vi "Working Point 2 Selection Dialog.vi"(7 "DisplayFilter":u8(ring)=7 items=["K_CHAN_R", "K_CHAN_W", "K_CHAN_RW", "K_CHAN_VOLT", "K_CHAN_FAULT", "K_ALL", "K_CUSTOM", "K_CHAN_R_VIS", "K_CHAN_W_VIS", "K_CHAN_RW_VIS", "K_CHAN_VOLT_VIS", "K_CHAN_FAULT_VIS"], 8 "error in (no error)":errorcluster, 9 "NIVS.System Definition Root":refnum<k24>, 10 "NodePaths":string[](array[string])) -> (0 "error out":errorcluster, 2 "Selected NodePaths":string[](array[string]))   [LabVIEW 2011]
doc: "Use this template to create a dialog box with event handling."
uses:
  NationalInstruments.VeriStand.SystemStorageUI
  NationalInstruments.VeriStand.SystemStorage
  <vilib>/NI Veristand/UI Controls/Single Node Browser/Net Event Data.ctl
  <vilib>/NI Veristand/UI Controls/Single Node Browser/Net Event.ctl
  <vilib>/NI Veristand/UI Controls/Single Node Browser/NI_VS UI Single Node Browser.lvlib
panel:
  in  "Y Value":refnum<k24>(container)
  in  "Cancel":bool
  in  "Ok":bool
  in  "X Index":refnum<k24>(container)
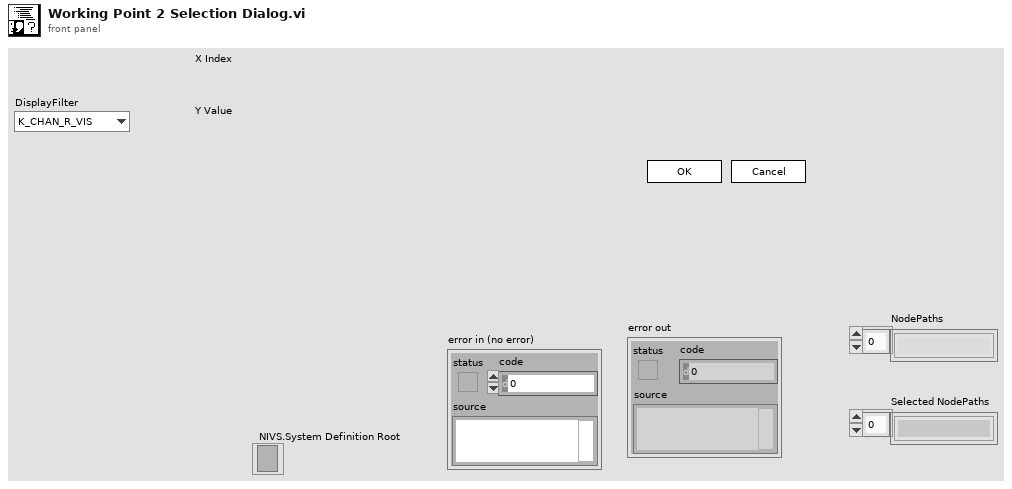
[diagram p1: front panel]
types:
  T1 = typedef "NI_VS UI Single Node Browser.lvlib/Callback Type.ctl" = cluster{"Net Callbacks":refnum<k27>[], "Event":refnum<user-event>}
  T2 = typedef "NI_VS UI Single Node Browser.lvlib/Node Ref.ctl" = refnum<k24>
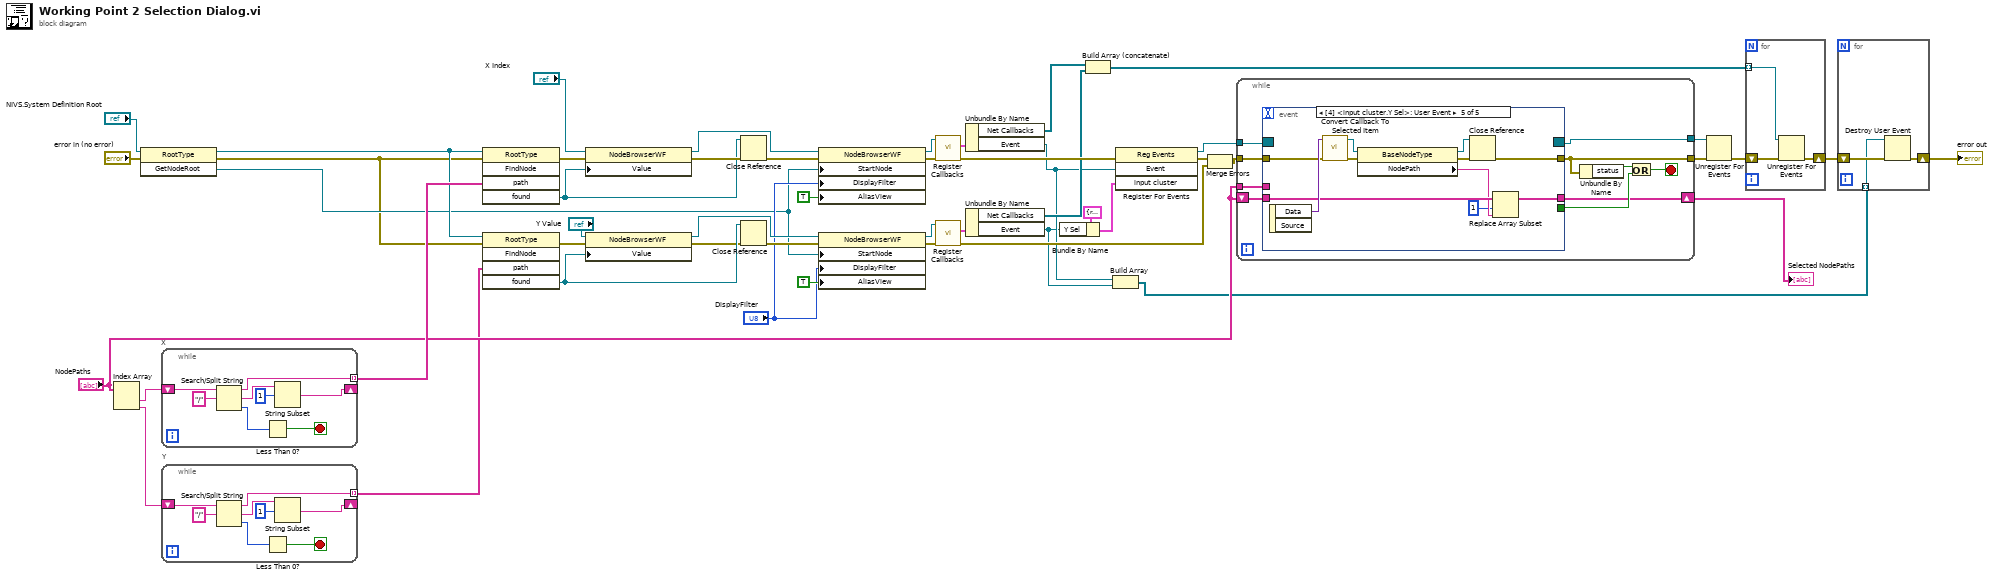
[diagram p0: block diagram]
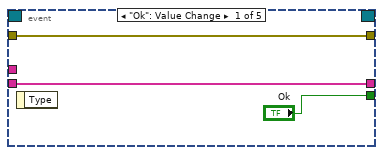
[diagram p2: hidden frame]
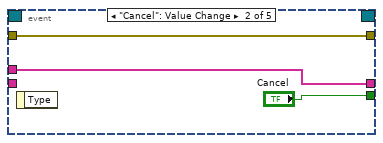
[diagram p3: hidden frame]
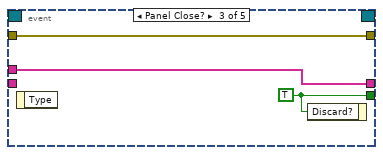
[diagram p4: hidden frame]
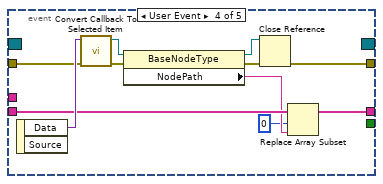
[diagram p5: hidden frame]
diagram:
  n1 = Index Array(array="NodePaths") -> (element #1=w30:string, element #2=w29:string)  [unwired: 2 in]
  n2 = invoke class="RootType" method="GetNodeRoot"(reference="NIVS.System Definition Root", error in="error in (no error)") -> (reference out=w18:refnum<k24>, error out=w14:errorcluster, "GetNodeRoot"=w15:refnum<k24>)  [unwired: 1 in]
  n3 = while "X" {
    tunnel: [w54] -> w36 mode=indexing
    shift-right: [w52] -> _
    shift-left: w30 -> [w58]
    stop <- w55 stop-if-true
    n4 = Search/Split String(string=w58, search string/char (-)="/") -> (substring before match=w54:string, match + rest of string=w53:string, offset of match=w56:i32)  [unwired: 1 in]
    n5 = Less Than 0?(x=w56) -> (x < 0?=w55:bool)
    n6 = String Subset(string=w53, offset (0)=1) -> (substring=w52:string)  [unwired: 1 in]
  }
  n7 = while "Y" {
    tunnel: [w62] -> w13 mode=indexing
    shift-right: [w60] -> _
    shift-left: w29 -> [w66]
    stop <- w63 stop-if-true
    n8 = Search/Split String(string=w66, search string/char (-)="/") -> (substring before match=w62:string, match + rest of string=w61:string, offset of match=w64:i32)  [unwired: 1 in]
    n9 = Less Than 0?(x=w64) -> (x < 0?=w63:bool)
    n10 = String Subset(string=w61, offset (0)=1) -> (substring=w60:string)  [unwired: 1 in]
  }
  n11 = invoke class="RootType" method="FindNode"(reference=w18, error in=w14, "path"=w36) -> (error out=w42:errorcluster, "found"=w37:refnum<k24>)  [unwired: 2 in, 3 out]
  n12 = invoke class="RootType" method="FindNode"(reference=w18, error in=w14, "path"=w13) -> (error out=w23:errorcluster, "found"=w26:refnum<k24>)  [unwired: 2 in, 3 out]
  n13 = property class="NodeBrowserWF"(reference="X Index", error in=w42, "Value"=w37) -> (reference out=w31:refnum<k24>, error out=w39:errorcluster)
  n14 = property class="NodeBrowserWF"(reference="Y Value", error in=w23, "Value"=w26) -> (reference out=w27:refnum<k24>, error out=w24:errorcluster)
  n15 = Close Reference(reference=w37, error in (no error)=w39) -> (error out=w38:errorcluster)
  n16 = Close Reference(reference=w26, error in (no error)=w24) -> (error out=w25:errorcluster)
  n17 = property class="NodeBrowserWF"(reference=w31, error in=w38, "StartNode"=w15, "DisplayFilter"="DisplayFilter", "AliasView"=TRUE) -> (reference out=w44:refnum<k24>, error out=w45:errorcluster)
  n18 = property class="NodeBrowserWF"(reference=w27, error in=w25, "StartNode"=w15, "DisplayFilter"="DisplayFilter", "AliasView"=TRUE) -> (reference out=w21:refnum<k24>, error out=w20:errorcluster)
  n19 = call <vilib>:"Register Callbacks.vi"("error in (no error)"=w45, "Single Node Browser"=w44) -> ("error out"=w50:errorcluster, "Callbacks"=w46:T1)  [unwired: 7 in, 1 out]
  n20 = call <vilib>:"Register Callbacks.vi"("error in (no error)"=w20, "Single Node Browser"=w21) -> ("error out"=w9:errorcluster, "Callbacks"=w19:T1)  [unwired: 7 in, 1 out]
  n21 = Unbundle By Name(w46) -> ("Net Callbacks"=w32:refnum<k27>[], "Event"=w4:refnum<user-event>)
  n22 = Unbundle By Name(w19) -> ("Net Callbacks"=w11:refnum<k27>[], "Event"=w3:refnum<user-event>)
  n23 = Bundle By Name(cluster=cluster{"Y Sel":refnum<user-event>} {"Y Sel"=refnum} ("input cluster"), "Y Sel"=w3) -> (w6:cluster{"Y Sel":refnum<user-event>})
  n24 = Build Array (concatenate)(w32, w11) -> (w12:refnum<k27>[])
  n25 = Build Array(w4, w3) -> (w2:refnum<user-event>[])
  n26 = register-events(error in=w50, w4, w6) -> (reference out=w49:refnum<event-registration>, error out=w40:errorcluster)  [unwired: 1 in]
  n27 = Merge Errors(w40, w9) -> (w10:errorcluster)
  n28 = while {
    tunnel: [w74] -> w35
    tunnel: w10 -> [w75]
    tunnel: w49 -> [w71]
    shift-right: [w70] -> w8
    shift-left: "NodePaths" -> [w69]
    tunnel: "NodePaths" -> [w68]
    tunnel: [w67] -> w34
    stop <- w73 stop-if-true
    n29 = event shown="[4] <input cluster.Y Sel>: User Event" {
      selector: w71 -> [_ _ _ _ _]
      dyn-events: [_ _ _ _ _] -> w67
      timeout: _ -> [_ _ _ _ _]
      tunnel: ["Ok" "Cancel" w85 _ _] -> w76
      tunnel: [w79 w81 w84 w94 w105] -> w74
      tunnel: w75 -> [w79 w81 w84 w95 w106]
      tunnel: [w77 w80 w83 w88 w99] -> w70
      tunnel: w69 -> [w77 _ _ w89 w100]
      tunnel: w68 -> [_ w80 w83 _ _]
      event "Ok": Value Change {
        n30 = event-data() -> ()  [unwired: 1 in, 1 out]
      }
      event "Cancel": Value Change {
        n31 = event-data() -> ()  [unwired: 1 in, 1 out]
      }
      event Panel Close? {
        w85 = TRUE ("Cancel")
        n32 = event-data() -> ()  [unwired: 1 in, 1 out]
        n33 = event-data("Discard?"=w85) -> ()  [unwired: 1 in, 1 out]
      }
      event User Event {
        n34 = event-data() -> ("Data"=w96:variant)  [unwired: 1 in, 1 out]
        n35 = call <vilib>:"Convert Callback To Selected Item.vi"("error in"=w95, "Data"=w96) -> ("error out"=w90:errorcluster, "Selected Item"=w93:T2)  [unwired: 8 in]
        n36 = property class="BaseNodeType"(reference=w93, error in=w90) -> (reference out=w92:T2, error out=w91:errorcluster, "NodePath"=w87:string)
        n37 = Close Reference(reference=w92, error in (no error)=w91) -> (error out=w94:errorcluster)
        n38 = Replace Array Subset(array=w89, new element=w87, index=0) -> (w88:string[])
      }
      event User Event {
        n39 = event-data() -> ("Data"=w107:variant)  [unwired: 1 in, 1 out]
        n40 = call <vilib>:"Convert Callback To Selected Item.vi"("error in"=w106, "Data"=w107) -> ("error out"=w101:errorcluster, "Selected Item"=w104:T2)  [unwired: 8 in]
        n41 = property class="BaseNodeType"(reference=w104, error in=w101) -> (reference out=w103:T2, error out=w102:errorcluster, "NodePath"=w98:string)
        n42 = Close Reference(reference=w103, error in (no error)=w102) -> (error out=w105:errorcluster)
        n43 = Replace Array Subset(array=w100, new element=w98, index=1) -> (w99:string[])
      }
    }
    n44 = Unbundle By Name(w74) -> ("status"=w72:bool)
    n45 = Or(x=w72, y=w76) -> (x .or. y?=w73:bool)
  }
  "Selected NodePaths" <- w8
  n46 = Unregister For Events(event registration refnum=w34, error in=w35) -> (error out=w33:errorcluster)
  n47 = for {
    tunnel: w12 -> [w109] mode=indexing
    shift-right: [w108] -> w5
    shift-left: w33 -> [w110]
    n48 = Unregister For Events(event registration refnum=w109, error in=w110) -> (error out=w108:errorcluster)
  }
  n49 = for {
    shift-right: [w112] -> w1
    shift-left: w5 -> [w113]
    tunnel: w2 -> [w111] mode=indexing
    n50 = Destroy User Event(user event=w111, error in=w113) -> (error out=w112:errorcluster)
  }
  "error out" <- w1
